vi "Test Suite Verdict Aggregates Results.vi"(8 "error in (no error)":errorcluster, 11 "Test Case In":refnum<class "LUnit Test Suite Tests.lvclass">) -> (0 "error out":errorcluster, 3 "Test Case Out":refnum<class "LUnit Test Suite Tests.lvclass">)   [LabVIEW 2020, in "LUnit Test Suite Tests.lvclass"]
uses:
  LUnit Test Suite Tests.lvclass
  C:/Program Files (x86)/National Instruments/LabVIEW 2020/vi.lib/Astemes/LUnit/Test Case.lvclass
  Test Case Test Double/Test Case Test Double.lvclass
  C:/Git/astemes-lunit/source/Core/LUnit Test Case/LUnit Test Case.lvclass
  <vilib>/Astemes/LUnit/Test Case.lvclass/Test Case.ctl
  b74e4934-f044-4222-b3dd-fc90e6c1bd4f.vi
  <vilib>/Astemes/LUnit/Palette/Pass.vi
  <vilib>/Astemes/LUnit/Palette/Fail.vi
  <vilib>/Astemes/LUnit/Compare Variants.vi
  <vilib>/Astemes/LUnit/Describe Comparison.vi
  <vilib>/Astemes/LUnit/Set Assertion Type.vi
  <vilib>/Astemes/LUnit/Add test result.vi
  <vilib>/Astemes/LUnit/Variant to string.vi
  <vilib>/Astemes/LUnit/LUnit Record Assertion Result.vi
  <vilib>/Astemes/LUnit/LUnit Aggregate Assertion Results.vi
  <vilib>/Astemes/LUnit/Method Result/LUnit Merge Status.vi
  <vilib>/Astemes/LUnit/LUnit Concatenate result strings.vi
  <vilib>/Utility/Data Type/Get Type Information.vi
  <vilib>/Utility/LVClass/Get LV Class Name.vi
  Core/LUnit Test Suite/LUnit Test Suite.lvclass
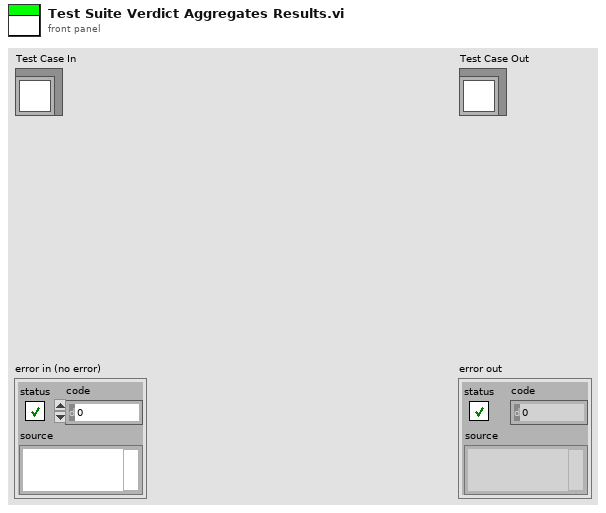
[diagram p1: front panel]
types:
  T1 = typedef "Result.lvlib/Result.ctl" = cluster{"Name":string, "Message":string, "Description":string, "Status":T2, "Result Type":T3, "Execution Time":dbl}
  T2 = typedef "Result.lvlib/Status.ctl" = enum16{"", "Passed", "Failed", "Error", "Skipped", "Setup Error", "Broken", "Teardown Error"}
  T3 = typedef "Result.lvlib/Type.ctl" = enum16{"Method", "Case", "Suite", "Pass", "Fail", "Skip", "Pass if", "Fail if", "Pass if Error", "Fail if Error", "Pass if Equal", "Fail if Equal"}
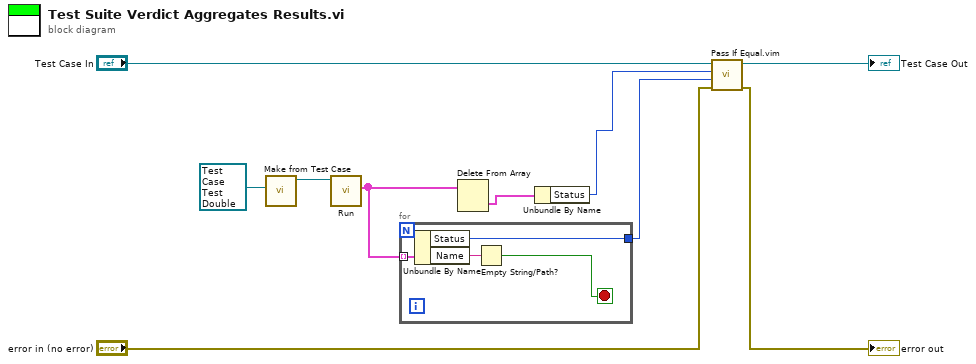
[diagram p0: block diagram]
diagram:
  n1 = call "Make from Test Case.vi"("LUnit Test Case"=refnum<class "Test Case Test Double.lvclass"> refnum ("LUnit Test Case V2 Test Double.lvclass")) -> ("LUnit Test Suite Out"=w6:refnum<class "LUnit Test Suite.lvclass">)  [unwired: 9 in, 1 out]
  n2 = call-dynamic "Run.vi"("LUnit Test Suite In"=w6) -> ("Results"=w4:T1[])  [unwired: 9 in, 1 out]
  n3 = for {
    tunnel: w4 -> [w14] mode=indexing
    tunnel: [w11] -> w3
    stop <- w12 stop-if-true
    n4 = Unbundle By Name(w14) -> ("Status"=w11:T2, "Name"=w13:string)
    n5 = Empty String/Path?(string/path=w13) -> (empty?=w12:bool)
  }
  n6 = Delete From Array(array=w4) -> (deleted portion=w2:T1)  [unwired: 2 in, 1 out]
  n7 = Unbundle By Name(w2) -> ("Status"=w1:T2)
  n8 = call "Pass If Equal.vim"("error in (no error)"="error in (no error)", "Actual"=w3, "Expected"=w1, "LUnit Test Case In"="Test Case In") -> ("error out"=→"error out":errorcluster, "LUnit Test Case Out"=→"Test Case Out":refnum<class "LUnit Test Suite Tests.lvclass">)  [unwired: 6 in]
